vi "Readable String.vi"(11 "Condition in":refnum<class "Condition.lvclass">) -> (2 "String":string)   [LabVIEW 2020, in "VolatusSeq.lvlib" / "Condition.lvclass"]
uses:
  Condition.lvclass
  Condition.lvclass/Condition.ctl
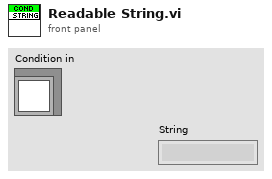
[diagram p1: front panel]
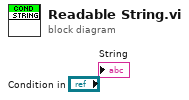
[diagram p0: block diagram]
diagram:
